vi "GLOBAL_STATE.vi"() -> ()   [LabVIEW 2017]
uses:
  libraryGcode/control/UartStatusBusy.ctl
panel:
  in  "State_Board_Control":T1=enum."Pos"
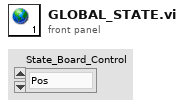
[diagram p1: front panel]
types:
  T1 = typedef "UartStatusBusy.ctl" = enum16{"Running", "Waiting", "Pos", "IDLE"}
diagram:
